vi "TankDriveCalc.vi"(10 "Drive Command Inputs":T1, 11 "Drive Sensor Inputs":T2) -> (3 "Drive Outputs":T3={"Front Left Speed"=-0.0325500651001302, "Front Right Speed"=0.03441006882013763, "Back Left Speed"=-0.0325500651001302, "Back Right Speed"=0.03441006882013763})   [LabVIEW 2012]
uses:
  Output_Wheel_Speeds.ctl
  Input_Sensors_Drive.ctl
  Input_Commands_Drive.ctl
panel:
  in  "Tipper alignment speed":dbl=-0.2
  in  "Tipper alignment time":u32
  in  "Drive.Max Drive Speed(Rotations/min)":dbl=1.0
  in  "P Right":dbl
  in  "I Right":dbl=0.01
  in  "D Right":dbl
  out "error out":errorcluster
  out "Waveform Chart":dbl[](graph)
  in  "Set PID":bool
  in  "D Left":dbl
  in  "I Left":dbl=0.01
  in  "P Left":dbl
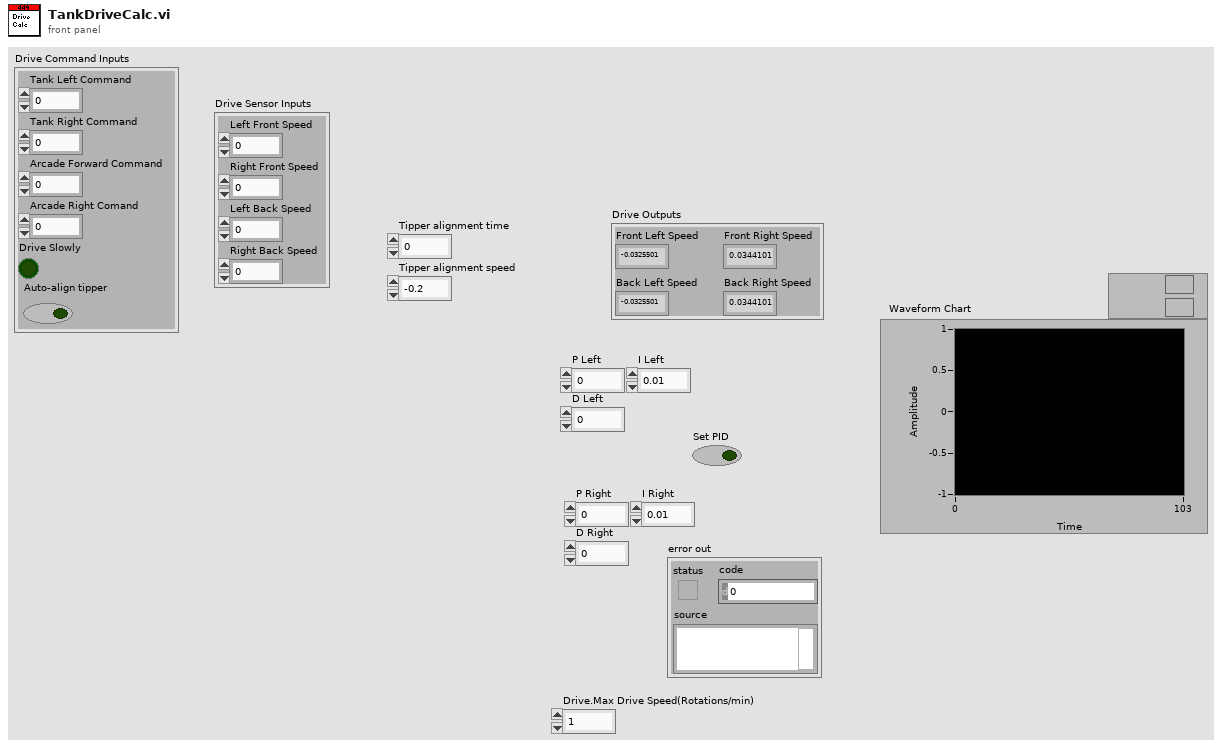
[diagram p1: front panel]
types:
  T1 = typedef "Input_Commands_Drive.ctl" = cluster{"Tank Left Command":dbl, "Tank Right Command":dbl, "Arcade Forward Command":dbl, "Arcade Right Comand":dbl, "Drive Slowly":bool, "Auto-align tipper":bool}
  T2 = typedef "Input_Sensors_Drive.ctl" = cluster{"Left Front Speed":dbl, "Right Front Speed":dbl, "Left Back Speed":dbl, "Right Back Speed":dbl}
  T3 = typedef "Output_Wheel_Speeds.ctl" = cluster{"Front Left Speed":dbl, "Front Right Speed":dbl, "Back Left Speed":dbl, "Back Right Speed":dbl}
  T4 = typedef "WPI_MotorControlDeviceRef.ctl" = cluster{"DeviceStatus":errorcluster, "Type":enum16{"PWM", "CAN"}, "PWM":cluster{"Digital Module":T5, "PWM Channel":T6, "DeadBand":T7}, "CAN":cluster{"Device Number":u8, "Control Mode":T8, "Semaphore":T9, "Max Vout":dbl}, "Invert":bool, "TransformRef":T10, "InvTransformRef":T10}
  T5 = typedef "FPGA_TypedefDigitalModule.ctl" = enum16{"Digital Module 1", "Digital Module 2"}
  T6 = typedef "FPGA_DIOPWMChannel.ctl" = enum8{"PWM 1", "PWM 2", "PWM 3", "PWM 4", "PWM 5", "PWM 6", "PWM 7", "PWM 8", "PWM 9", "PWM 10", "Invalid"}
  T7 = typedef "WPI_PWMDeadband.ctl" = cluster{"Name":string, "maxPositivePwm":i32, "minPositivePwm":i32, "centerPwm":i32, "maxNegativePwm":i32, "minNegativePwm":i32, "angularRange":u16}
  T8 = typedef "WPI_CANJaguar_ControlMode.ctl" = enum8{"Percent VBus", "Current", "Speed", "Position", "Voltage"}
  T9 = typedef "Semaphore RefNum" = refnum<k1>
  T10 = typedef "WPI_PWMTransform_ConPane.ctl" = refnum<vi>
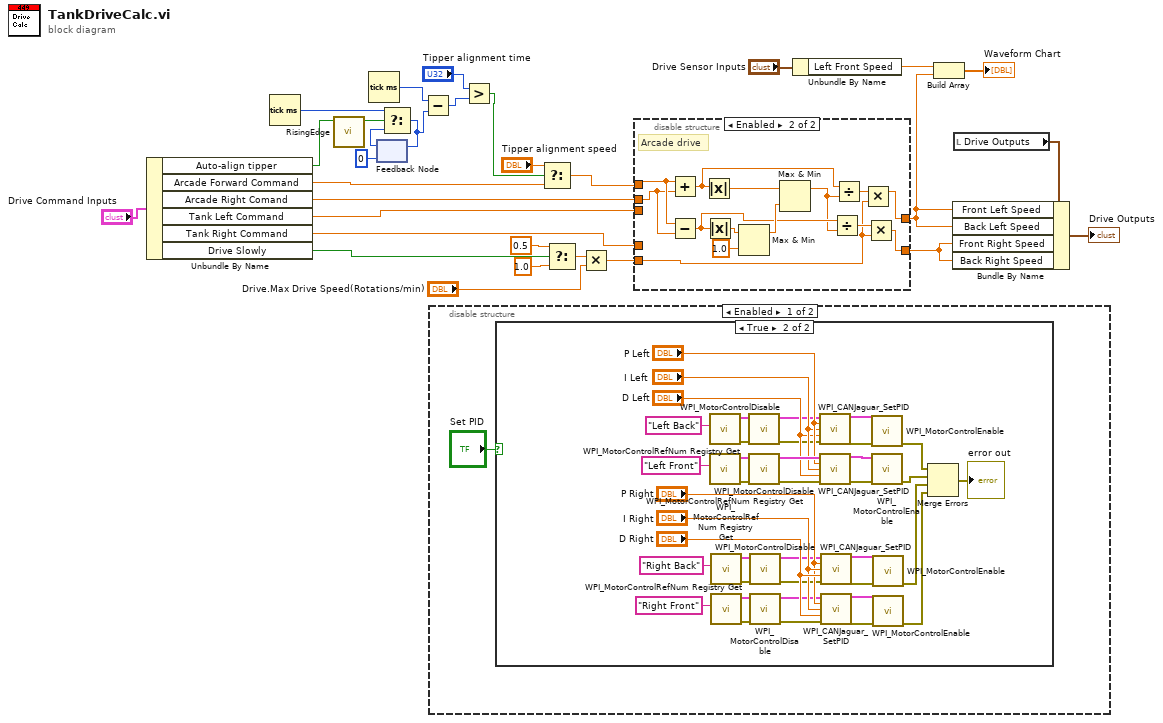
[diagram p0: block diagram]
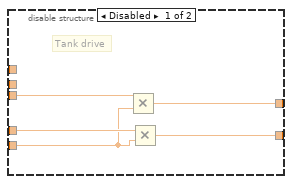
[diagram p4: hidden frame]
diagram:
  n1 = Unbundle By Name("Drive Command Inputs") -> ("Auto-align tipper"=w13:bool, "Arcade Forward Command"=w4:dbl, "Arcade Right Comand"=w25:dbl, "Tank Left Command"=w27:dbl, "Tank Right Command"=w28:dbl, "Drive Slowly"=w19:bool)
  n2 = Tick Count (ms)() -> (millisecond timer value=w10:u32)
  n3 = call "RisingEdge.vi"("BooleanIn"=w13) -> ("BooleanOut"=w12:bool)  [unwired: 10 in]
  n4 = Tick Count (ms)() -> (millisecond timer value=w8:u32)
  n5 = feedback #1(u32 0 ("millisecond timer value")) -> (w11:u32)
  n6 = Select(t=w10, s=w12, f=w11) -> (s? t:f=w9:u32)
  n7 = feedback-in #1(w9) -> ()
  n8 = Subtract(x=w8, y=w9) -> (x-y=w6:u32)
  n9 = disable-structure shown="Enabled" {
    frame Enabled {
      n10 = case shown="True" "Set PID" {
        frame False {
        }
        frame True {
          n11 = call <vilib>:"WPI_MotorControlRefNum Registry Get.vi"("refnum name"="Left Back") -> ("error out"=w51:errorcluster, "MotorControlDevRef"=w50:T4)  [unwired: 9 in]
          n12 = call <vilib>:"WPI_MotorControlRefNum Registry Get.vi"("refnum name"="Left Front") -> ("error out"=w65:errorcluster, "MotorControlDevRef"=w66:T4)  [unwired: 9 in]
          n13 = call <vilib>:"WPI_MotorControlRefNum Registry Get.vi"("refnum name"="Right Back") -> ("error out"=w33:errorcluster, "MotorControlDevRef"=w34:T4)  [unwired: 9 in]
          n14 = call <vilib>:"WPI_MotorControlRefNum Registry Get.vi"("refnum name"="Right Front") -> ("error out"=w44:errorcluster, "MotorControlDevRef"=w43:T4)  [unwired: 9 in]
          n15 = call <vilib>:"WPI_MotorControlDisable.vi"("error in (no error)"=w51, "MotorControlDevRef"=w50) -> ("error out"=w48:errorcluster, "MotorControlDevRef"=w49:T4)  [unwired: 8 in]
          n16 = call <vilib>:"WPI_MotorControlDisable.vi"("error in (no error)"=w65, "MotorControlDevRef"=w66) -> ("error out"=w68:errorcluster, "MotorControlDevRef"=w67:T4)  [unwired: 8 in]
          n17 = call <vilib>:"WPI_MotorControlDisable.vi"("error in (no error)"=w33, "MotorControlDevRef"=w34) -> ("error out"=w36:errorcluster, "MotorControlDevRef"=w35:T4)  [unwired: 8 in]
          n18 = call <vilib>:"WPI_MotorControlDisable.vi"("error in (no error)"=w44, "MotorControlDevRef"=w43) -> ("error out"=w41:errorcluster, "MotorControlDevRef"=w42:T4)  [unwired: 8 in]
          n19 = call <vilib>:"WPI_CANJaguar_SetPID.vi"("CAN Jaguar Ref"=w49, "P"="P Left", "I"="I Left", "D"="D Left", "error in (no error)"=w48) -> ("CAN Jaguar Ref Out"=w47:T4, "error out"=w46:errorcluster)  [unwired: 9 in]
          n20 = call <vilib>:"WPI_CANJaguar_SetPID.vi"("CAN Jaguar Ref"=w67, "P"="P Left", "I"="I Left", "D"="D Left", "error in (no error)"=w68) -> ("CAN Jaguar Ref Out"=w69:T4, "error out"=w70:errorcluster)  [unwired: 9 in]
          n21 = call <vilib>:"WPI_CANJaguar_SetPID.vi"("CAN Jaguar Ref"=w35, "P"="P Right", "I"="I Right", "D"="D Right", "error in (no error)"=w36) -> ("CAN Jaguar Ref Out"=w37:T4, "error out"=w38:errorcluster)  [unwired: 9 in]
          n22 = call <vilib>:"WPI_CANJaguar_SetPID.vi"("CAN Jaguar Ref"=w42, "P"="P Right", "I"="I Right", "D"="D Right", "error in (no error)"=w41) -> ("CAN Jaguar Ref Out"=w40:T4, "error out"=w39:errorcluster)  [unwired: 9 in]
          n23 = call <vilib>:"WPI_MotorControlEnable.vi"("error in (no error)"=w46, "CAN Jaguar Ref"=w47) -> ("error out"=w63:errorcluster)  [unwired: 8 in, 1 out]
          n24 = call <vilib>:"WPI_MotorControlEnable.vi"("error in (no error)"=w70, "CAN Jaguar Ref"=w69) -> ("error out"=w62:errorcluster)  [unwired: 8 in, 1 out]
          n25 = call <vilib>:"WPI_MotorControlEnable.vi"("error in (no error)"=w38, "CAN Jaguar Ref"=w37) -> ("error out"=w61:errorcluster)  [unwired: 8 in, 1 out]
          n26 = call <vilib>:"WPI_MotorControlEnable.vi"("error in (no error)"=w39, "CAN Jaguar Ref"=w40) -> ("error out"=w60:errorcluster)  [unwired: 8 in, 1 out]
          n27 = Merge Errors(w63, w62, w61, w60) -> (→"error out":errorcluster)
        }
      }
    }
    frame Disabled {
    }
  }
  n28 = Greater?(x="Tipper alignment time", y=w6) -> (0:w2:bool)
  n29 = Select(t="Tipper alignment speed", s=w2, f=w4) -> (s? t:f=w3:dbl)
  n30 = Select(t=0.5, s=w19, f=1.0) -> (s? t:f=w16:dbl)
  n31 = Multiply(x=w16, y="Drive.Max Drive Speed(Rotations/min)") -> (x*y=w14:dbl)
  n32 = disable-structure shown="Enabled" {
    disable-tunnel: w28 -> [w75 _]
    disable-tunnel: w14 -> [w74 w76]
    disable-tunnel: w27 -> [w73 _]
    disable-tunnel: [w72 w79] -> w23
    disable-tunnel: [w71 w78] -> w26
    disable-tunnel: w25 -> [_ w88]
    disable-tunnel: w3 -> [_ w89]
    frame Disabled {
      # "Tank drive"
      n33 = Multiply(x=w73, y=w74) -> (x*y=w72:dbl)
      n34 = Multiply(x=w75, y=w74) -> (x*y=w71:dbl)
    }
    frame Enabled {
      # "Arcade drive"
      n35 = Add(x=w89, y=w88) -> (x+y=w83:dbl)
      n36 = Subtract(x=w89, y=w88) -> (x-y=w82:dbl)
      n37 = Absolute Value(x=w83) -> (abs(x)=w87:dbl)
      n38 = Absolute Value(x=w82) -> (abs(x)=w86:dbl)
      n39 = Max & Min(x=w86, y=1.0) -> (max(x,y)=w84:dbl)  [unwired: 1 out]
      n40 = Max & Min(x=w87, y=w84) -> (max(x,y)=w81:dbl)  [unwired: 1 out]
      n41 = Divide(x=w82, y=w81) -> (x/y=w77:dbl)
      n42 = Divide(x=w83, y=w81) -> (x/y=w80:dbl)
      n43 = Multiply(x=w80, y=w76) -> (x*y=w79:dbl)
      n44 = Multiply(x=w77, y=w76) -> (x*y=w78:dbl)
    }
  }
  n45 = Unbundle By Name("Drive Sensor Inputs") -> ("Left Front Speed"=w21:dbl)
  n46 = Build Array(w21, w23) -> (→"Waveform Chart":dbl[])
  n47 = local read "Drive Outputs"() -> (w29:T3)
  n48 = Bundle By Name(cluster=w29, "Front Left Speed"=w23, "Back Left Speed"=w23, "Front Right Speed"=w26, "Back Right Speed"=w26) -> (→"Drive Outputs":T3)
